vi "grSim Robot Command.vi"(7 "YellowTeam?":bool=TRUE, 9 "Array In":u8[](array[numeric]), 10 "FIRASim?":bool=TRUE, 11 "Robots":T1) -> (1 "Array":u8[](array[numeric]))   [LabVIEW 2023]
uses:
  Convert AI Robot to Robot Command Folder/grSim/grSim Robot Command.ctl
  MessageAI_State Folder/Varint Encoder uint32.vi
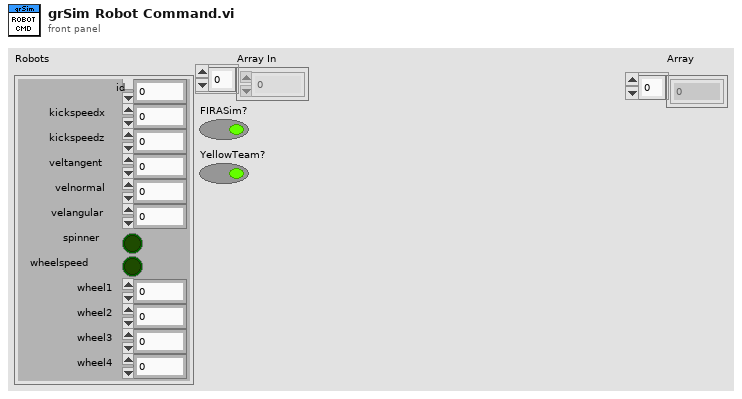
[diagram p1: front panel]
types:
  T1 = typedef "grSim Robot Command.ctl" = cluster{"id":u32, "kickspeedx":sgl, "kickspeedz":sgl, "veltangent":sgl, "velnormal":sgl, "velangular":sgl, "spinner":bool, "wheelspeed":bool, "wheel1":sgl, "wheel2":sgl, "wheel3":sgl, "wheel4":sgl}
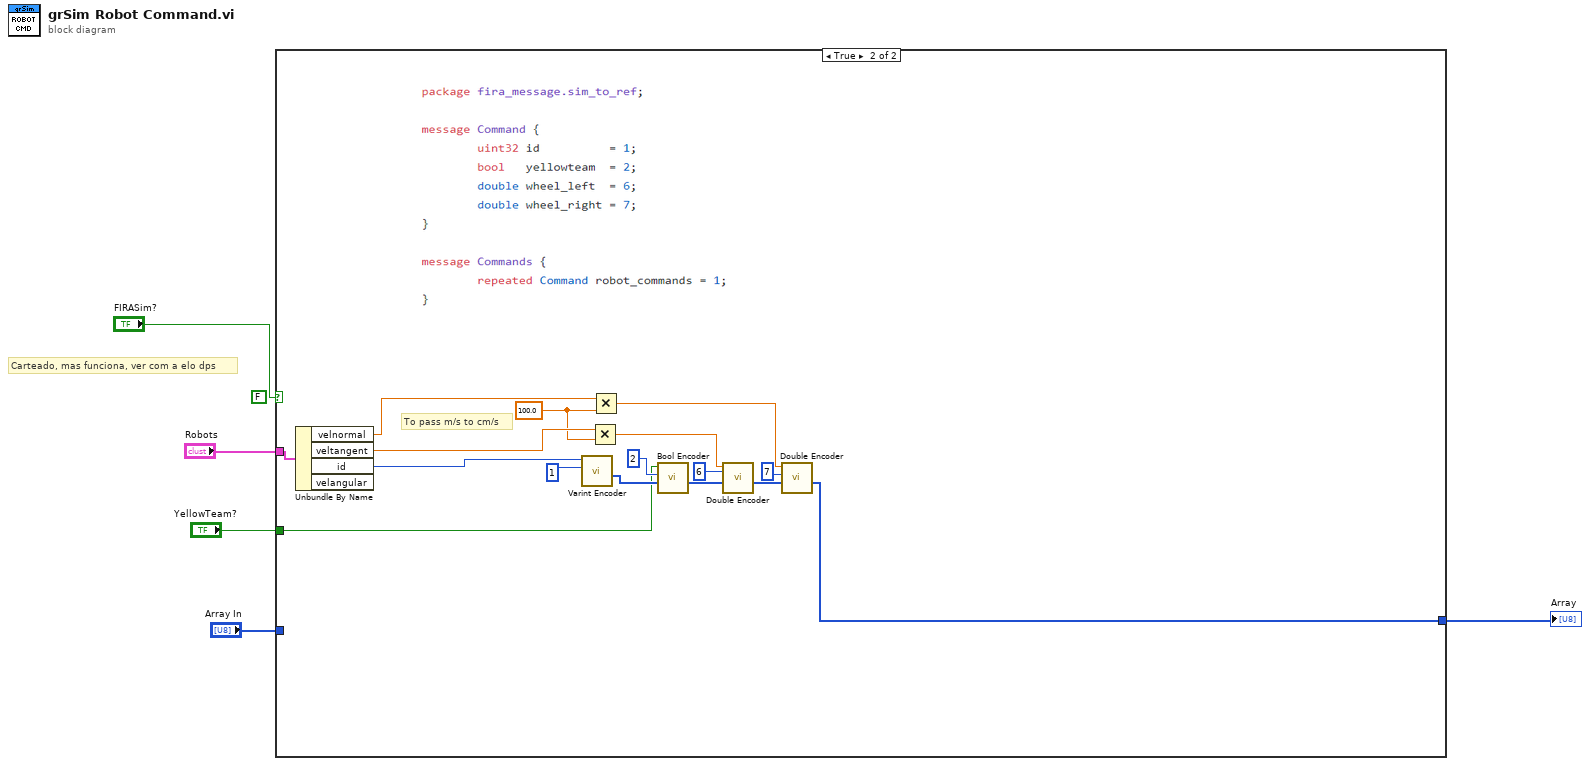
[diagram p0: block diagram]
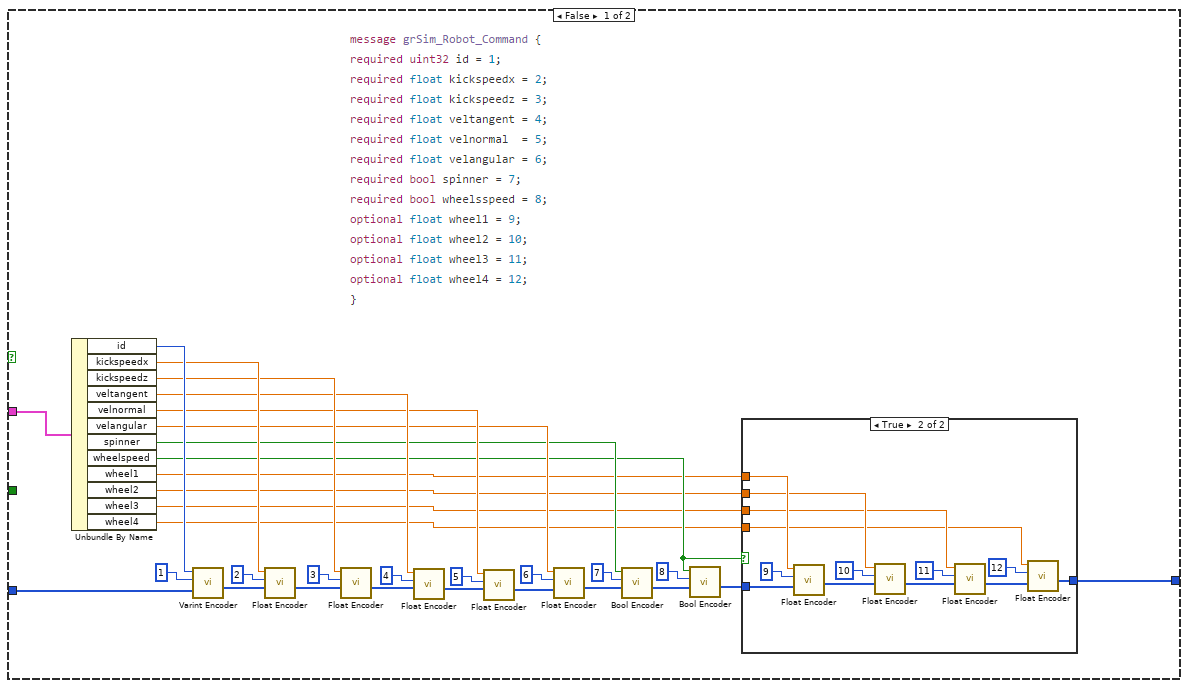
[diagram p2: hidden frame]
diagram:
  (unwired) FALSE
  # "Carteado, mas funciona, ver com a elo dps"
  n1 = case shown="True" "FIRASim?" {
    tunnel: "Robots" -> [w36 w58]
    tunnel: [w7 w59] -> w4
    tunnel: "YellowTeam?" -> [_ w56]
    tunnel: "Array In" -> [w6 _]
    frame False {
      n2 = Unbundle By Name(w36) -> ("id"=w35:u32, "kickspeedx"=w31:sgl, "kickspeedz"=w22:sgl, "veltangent"=w21:sgl, "velnormal"=w20:sgl, "velangular"=w19:sgl, "spinner"=w14:bool, "wheelspeed"=w13:bool, "wheel1"=w11:sgl, "wheel2"=w10:sgl, "wheel3"=w9:sgl, "wheel4"=w8:sgl)
      n3 = call-poly "Varint Encoder.vi"("Array In"=w6, "Key"=u32 1, "Value"=w35) -> ("Array"=w33:u8[])  [unwired: 8 in]
      n4 = call "Float Encoder.vi"("Array In"=w33, "Key"=u32 2, "Value"=w31) -> ("Array"=w26:u8[])  [unwired: 8 in]
      n5 = call "Float Encoder.vi"("Array In"=w26, "Key"=u32 3, "Value"=w22) -> ("Array"=w25:u8[])  [unwired: 8 in]
      n6 = call "Float Encoder.vi"("Array In"=w25, "Key"=u32 4, "Value"=w21) -> ("Array"=w24:u8[])  [unwired: 8 in]
      n7 = call "Float Encoder.vi"("Array In"=w24, "Key"=u32 5, "Value"=w20) -> ("Array"=w23:u8[])  [unwired: 8 in]
      n8 = call "Float Encoder.vi"("Array In"=w23, "Key"=u32 6, "Value"=w19) -> ("Array"=w18:u8[])  [unwired: 8 in]
      n9 = call "Bool Encoder.vi"("Array In"=w18, "Key"=u32 7, "Value"=w14) -> ("Array"=w16:u8[])  [unwired: 8 in]
      n10 = call "Bool Encoder.vi"("Array In"=w16, "Key"=u32 8, "Value"=w13) -> ("Array"=w12:u8[])  [unwired: 8 in]
      n11 = case shown="True" w13 {
        tunnel: w12 -> [w37 w49]
        tunnel: w11 -> [_ w42]
        tunnel: w10 -> [_ w41]
        tunnel: w9 -> [_ w40]
        tunnel: w8 -> [_ w39]
        tunnel: [w37 w38] -> w7
        frame False {
        }
        frame True {
          n12 = call "Float Encoder.vi"("Array In"=w49, "Key"=u32 9, "Value"=w42) -> ("Array"=w45:u8[])  [unwired: 8 in]
          n13 = call "Float Encoder.vi"("Array In"=w45, "Key"=u32 10, "Value"=w41) -> ("Array"=w44:u8[])  [unwired: 8 in]
          n14 = call "Float Encoder.vi"("Array In"=w44, "Key"=u32 11, "Value"=w40) -> ("Array"=w43:u8[])  [unwired: 8 in]
          n15 = call "Float Encoder.vi"("Array In"=w43, "Key"=u32 12, "Value"=w39) -> ("Array"=w38:u8[])  [unwired: 8 in]
        }
      }
    }
    frame True {
      w52 = 100.0
      # "To pass m/s to cm/s"
      n16 = Unbundle By Name(w58) -> ("velnormal"=w55:sgl, "veltangent"=w53:sgl, "id"=w57:u32)  [unwired: 1 out]
      n17 = call-poly "Varint Encoder.vi"("Key"=u32 1, "Value"=w57) -> ("Array"=w65:u8[])  [unwired: 9 in]
      n18 = Multiply(x=w53, y=w52) -> (x*y=w51:dbl)
      n19 = Multiply(x=w55, y=w52) -> (x*y=w54:dbl)
      n20 = call "Bool Encoder.vi"("Array In"=w65, "Key"=u32 2, "Value"=w56) -> ("Array"=w63:u8[])  [unwired: 8 in]
      n21 = call "Double Encoder.vi"("Array In"=w63, "Key"=u32 6, "Value"=w51) -> ("Array"=w62:u8[])  [unwired: 8 in]
      n22 = call "Double Encoder.vi"("Array In"=w62, "Key"=u32 7, "Value"=w54) -> ("Array"=w59:u8[])  [unwired: 8 in]
    }
  }
  "Array" <- w4
